vi "Aula 2.vi"() -> ()   [LabVIEW 2020]
panel:
  in  "Item B":u8
  out "C = A + B":u8
  in  "Item A":u8
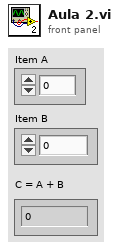
[diagram p1: front panel]
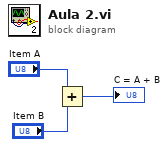
[diagram p0: block diagram]
diagram:
  n1 = Add(x="Item A", y="Item B") -> (x+y=→"C = A + B":u8)
